vi "Convert Bits to Genealogy.vi"(8 "error in (no error)":errorcluster, 10 "SN ASCII":i32[](array[numeric])=[81, 77, 67, 2200123], 11 "PN 64Base":u8[](array[numeric])=[53, 52, 52, 52, 52, 52, 52, 53]) -> (0 "error out":errorcluster, 2 "SN out":string="QMC2200123", 3 "PN out":string="10-000001")   [LabVIEW 2019, in "Measuremtn Abstraction.lvlib"]
uses:
  Measuremtn Abstraction.lvlib
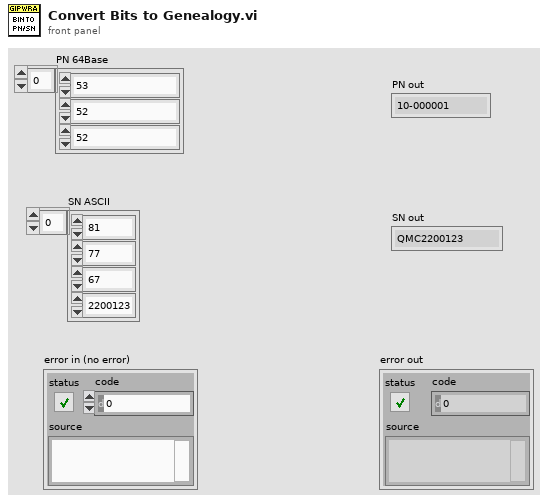
[diagram p1: front panel]
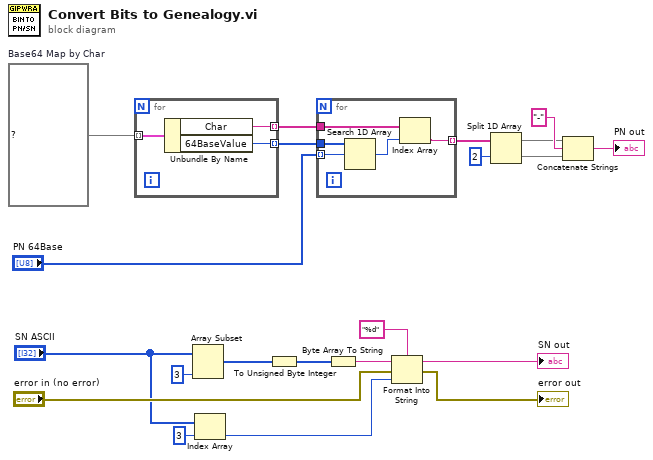
[diagram p0: block diagram]
diagram:
  w16 = map{string, u8} {"+"=62, "/"=63, "0"=52, "1"=53, "2"=54, "3"=55, "4"=56, "5"=57, "6"=58, "7"=59, "8"=60, "9"=61, "A"=0, "B"=1, "C"=2, "D"=3, "E"=4, "F"=5, "G"=6, "H"=7, "I"=8, "J"=9, "K"=10, "L"=11, "M"=12, "N"=13, "O"=14, "P"=15, "Q"=16, "R"=17, "S"=18, "T"=19, "U"=20, "V"=21, "W"=22, "X"=23, "Y"=24, "Z"=25, "a"=26, "b"=27, "c"=28, "d"=29, "e"=30, "f"=31, "g"=32, "h"=33, "i"=34, "j"=35, "k"=36, "l"=37, "m"=38, "n"=39, "o"=40, "p"=41, "q"=42, "r"=43, "s"=44, "t"=45, "u"=46, "v"=47, "w"=48, "x"=49, "y"=50, "z"=51}  # Base64 Map by Char
  n1 = for {
    tunnel: w16 -> [w24] mode=indexing
    tunnel: [w23] -> w15 mode=indexing
    tunnel: [w22] -> w13 mode=indexing
    n2 = Unbundle By Name(w24) -> ("Char"=w22:string, "64BaseValue"=w23:u8)
  }
  n3 = Array Subset(array="SN ASCII", length=3) -> (w5:i32[])  [unwired: 1 in]
  n4 = Index Array(array="SN ASCII", index=3) -> (element=w1:i32)
  n5 = To Unsigned Byte Integer(number=w5) -> (unsigned 8bit integer=w4:u8[])
  n6 = for {
    tunnel: w15 -> [w29]
    tunnel: "PN 64Base" -> [w28] mode=indexing
    tunnel: w13 -> [w27]
    tunnel: [w25] -> w9 mode=indexing
    n7 = Search 1D Array(1D array=w29, element=w28) -> (index of element=w26:i32)  [unwired: 1 in]
    n8 = Index Array(array=w27, index=w26) -> (element=w25:string)
  }
  n9 = Byte Array To String(unsigned byte array=w4) -> (string=w21:string)
  n10 = Format Into String(format string="%d", initial string=w21, error in="error in (no error)", w1) -> (resulting string=→"SN out":string, error out=→"error out":errorcluster)
  n11 = Split 1D Array(array=w9, index=2) -> (first subarray=w8:string[], second subarray=w7:string[])
  n12 = Concatenate Strings(w8, "-" ("string"), w7) -> (→"PN out":string)
